vi "init_lasers.vi"(7 "488 pulsed":bool, 9 "594 nm voltage":dbl, 11 "488 nm channel parameters":T1={"voltage"=0.0, "frequency"=0.0, "duty cycle"=0.0, "sample rate"=1000.0}) -> (0 "error out":errorcluster, 2 "current data":cluster{"[0]":dbl, "[1]":dbl}, 3 "task out":refnum<k21>)   [LabVIEW 2025]
uses:
  channel parameters cluster.ctl
  <vilib>/DAQmx/write.llb/DAQmx Write (Analog 1D Wfm NChan NSamp).vi
  <vilib>/DAQmx/create/channels.llb/DAQmx Create Channel (AO-Voltage-Basic).vi
  <vilib>/DAQmx/configure/timing.llb/DAQmx Timing (Sample Clock).vi
  <vilib>/DAQmx/miscellaneous.llb/DAQmx Fill In Error Info.vi
  <resource>/objmgr/daqmx.rc
  <vilib>/DAQmx/write.llb/DAQmx Write (Analog 1D DBL NChan 1Samp).vi
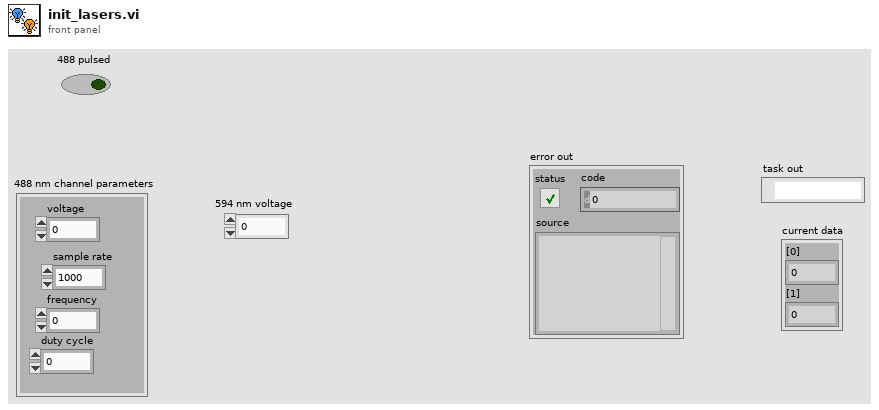
[diagram p1: front panel]
types:
  T1 = typedef "channel parameters cluster.ctl" = cluster{"voltage":dbl, "frequency":dbl, "duty cycle":dbl, "sample rate":dbl}
  T2 = cluster{" waveforms out[0]":waveform(dbl), " waveforms out[1]":waveform(dbl)}
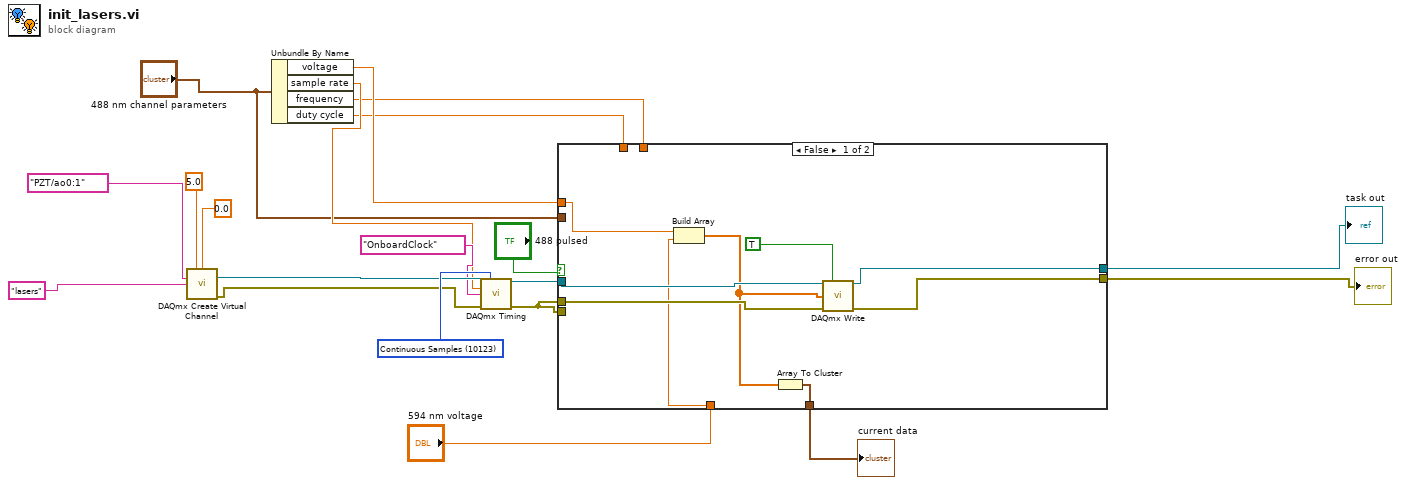
[diagram p0: block diagram]
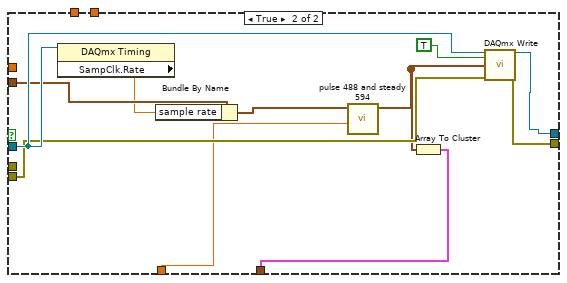
[diagram p2: hidden frame]
diagram:
  w18 = 10123 items=["Finite Samples"=10178, "Continuous Samples"=10123, "Hardware Timed Single Point"=12522] ("SampQuant.SampMode")
  n1 = call-poly <vilib>:"DAQmx Create Virtual Channel.vi"("maximum value"=5.0, "minimum value"=0.0, "physical channels"=tag "PZT/ao0:1", "name to assign"="lasers") -> ("task out"=w16:refnum<k21>, "error out"=w17:errorcluster)  [unwired: 10 in]
  n2 = Unbundle By Name("488 nm channel parameters") -> ("voltage"=w12:dbl, "sample rate"=w11:dbl, "frequency"=w9:dbl, "duty cycle"=w10:dbl)
  n3 = call-poly <vilib>:"DAQmx Timing.vi"("task/channels in"=w16, "sample mode"=w18, "rate"=w11, "source"=tag "OnboardClock", "error in"=w17) -> ("task out"=w13:refnum<k21>, "error out"=w6:errorcluster)  [unwired: 9 in]
  n4 = case shown="False" "488 pulsed" {
    tunnel: w13 -> [w29 w40]
    tunnel: w6 -> [w28 _]
    tunnel: w12 -> [w23 _]
    tunnel: w10 -> [_ _]
    tunnel: w9 -> [_ _]
    tunnel: w6 -> [_ w39]
    tunnel: [w26 w38] -> w5
    tunnel: [w25 w37] -> w4
    tunnel: "594 nm voltage" -> [w22 w33]
    tunnel: [w24 w35] -> w2
    tunnel: "488 nm channel parameters" -> [_ w32]
    frame False {
      n5 = Build Array(w23, w22) -> (w21:dbl[])
      n6 = Array To Cluster(array=w21) -> (cluster=w24:cluster{"[0]":dbl, "[1]":dbl})
      n7 = call-poly <vilib>:"DAQmx Write.vi"("task/channels in"=w29, "auto start"=TRUE, "data"=w21, "error in"=w28) -> ("task out"=w26:refnum<k21>, "error out"=w25:errorcluster)  [unwired: 9 in, 1 out]
    }
    frame True {
      n8 = property class="DAQmx Timing"(reference=w40) -> ("SampClk.Rate"=w30:dbl)  [unwired: 1 in, 2 out]
      n9 = Bundle By Name(cluster=w32, "sample rate"=w30) -> (w31:T1)
      n10 = call "pulse 488 and steady 594.vi"("594 amplitude"=w33, "488 nm channel parameters"=w31) -> ("waveforms out"=w34:waveform(dbl)[])  [unwired: 9 in]
      n11 = Array To Cluster(array=w34) -> (cluster=w35:T2)
      n12 = call-poly <vilib>:"DAQmx Write.vi"("task/channels in"=w40, "auto start"=TRUE, "data"=w34, "error in"=w39) -> ("task out"=w38:refnum<k21>, "error out"=w37:errorcluster)  [unwired: 9 in, 1 out]
    }
  }
  "error out" <- w4
  "task out" <- w5
  "current data" <- w2
